vi "generate default name.vi"(11 "Info":T1={"Make"="Canon\u0000", "Model"="Canon PowerShot A495\u0000", "Orientation"=0, "Date"=timestamp(0 s since 1904-01-01), "Width"=0, "Height"=0, "Square?"=FALSE, "File Name"="Canon\u0000", "Extension"="Canon\u0000", "Valid?"=FALSE, "Path"=path "", "size"=0, "No Ext?"=FALSE, "prefix?"=FALSE, "Tag"="", "Name Type"=enum."Event Sufix", "Projection Type"="Canon\u0000"}) -> (1 "Model":string, 3 "default name":string)   [LabVIEW 2023, in "File Classes.lvlib" / "Picture File.lvclass"]
uses:
  Picture File.lvclass
  Controls/exif data cluster.ctl
  Controls/rename type enum.ctl
  <vilib>/gmath/NI_Gmath.lvlib
  File Classes.lvlib
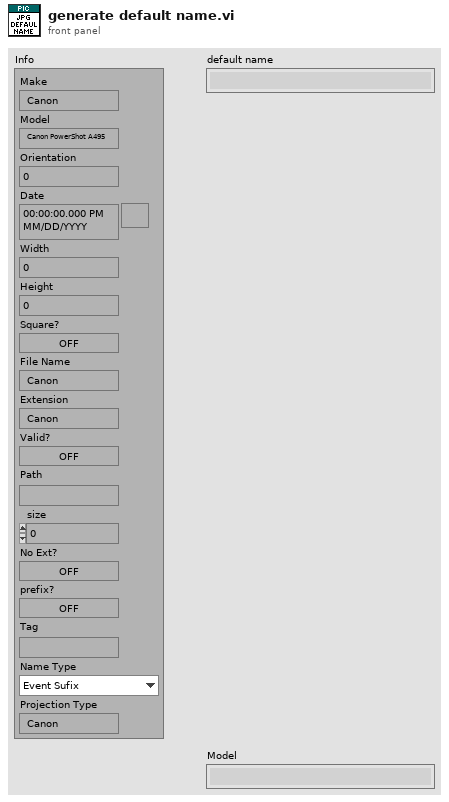
[diagram p1: front panel]
types:
  T1 = typedef "File Classes.lvlib/exif data cluster.ctl" = cluster{"Make":string, "Model":string, "Orientation":u16, "Date":timestamp, "Width":u16, "Height":u16, "Square?":bool, "File Name":string, "Extension":string, "Valid?":bool, "Path":path, "size":i64, "No Ext?":bool, "prefix?":bool, "Tag":string, "Name Type":T2, "Projection Type":string}
  T2 = typedef "File Classes.lvlib/rename type enum.ctl" = enum16{"Date & Time (Default)", "Model Sufix", "Event Sufix", "Model & Event Sufix"}
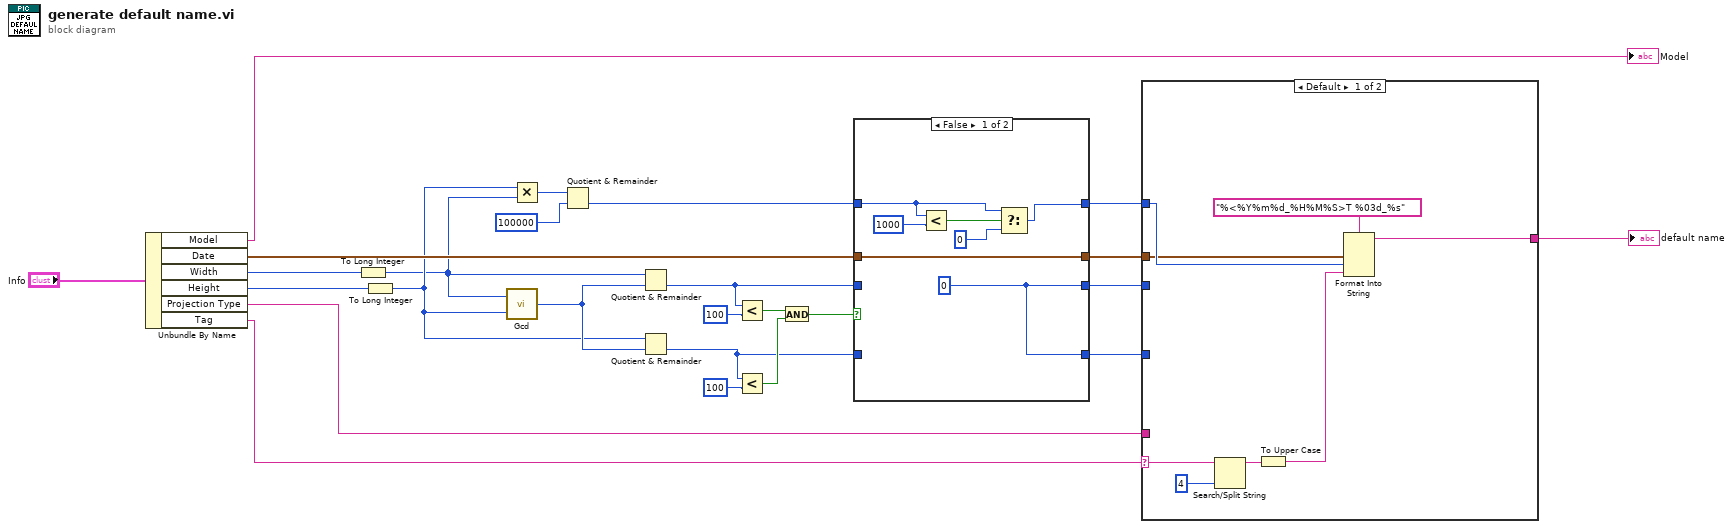
[diagram p0: block diagram]
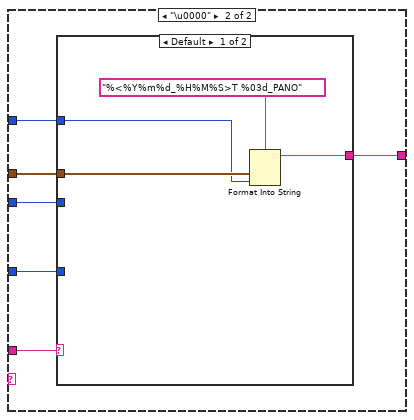
[diagram p2: hidden frame]
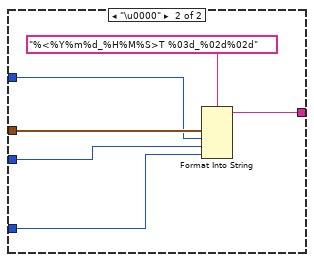
[diagram p3: hidden frame]
diagram:
  n1 = Unbundle By Name("Info") -> ("Model"=→"Model":string, "Date"=w23:timestamp, "Width"=w21:u16, "Height"=w20:u16, "Projection Type"=w2:string, "Tag"=w1:string)
  n2 = To Long Integer(number=w21) -> (32bit integer=w3:i32)
  n3 = To Long Integer(number=w20) -> (32bit integer=w12:i32)
  n4 = call <vilib>:"Gcd.vi"("y"=w12, "x"=w3) -> ("gcd(x,y)"=w15:i32)
  n5 = Multiply(x=w12, y=w3) -> (x*y=w14:i32)
  n6 = Quotient & Remainder(x=w14, y=100000) -> (floor(x/y)=w10:i32)  [unwired: 1 out]
  n7 = Quotient & Remainder(x=w3, y=w15) -> (floor(x/y)=w8:i32)  [unwired: 1 out]
  n8 = Quotient & Remainder(x=w12, y=w15) -> (floor(x/y)=w6:i32)  [unwired: 1 out]
  n9 = Less?(x=w8, y=100) -> (x < y?=w19:bool)
  n10 = Less?(x=w6, y=100) -> (x < y?=w18:bool)
  n11 = And(x=w19, y=w18) -> (x .and. y?=w11:bool)
  n12 = case shown="False" w11 {
    tunnel: [w29 w33] -> w4
    tunnel: w10 -> [w28 w33]
    tunnel: [w32 w34] -> w9
    tunnel: w23 -> [w32 w34]
    tunnel: [w27 w36] -> w5
    tunnel: w8 -> [_ w36]
    tunnel: [w27 w35] -> w7
    tunnel: w6 -> [_ w35]
    frame False {
      w27 = 0
      n13 = Less?(x=w28, y=1000) -> (x < y?=w30:bool)
      n14 = Select(t=w28, s=w30, f=0) -> (s? t:f=w29:i32)
    }
    frame True {
    }
  }
  n15 = case shown="Default" w1 {
    selector: w1 -> [w40 _]
    tunnel: [w41 w50] -> w25
    tunnel: w9 -> [w42 w49]
    tunnel: w7 -> [_ w48]
    tunnel: w5 -> [_ w47]
    tunnel: w4 -> [w43 w46]
    tunnel: w2 -> [_ w45]
    frame Default {
      n16 = Search/Split String(string=w40, offset (0)=4) -> (substring before match=w38:string)  [unwired: 1 in, 2 out]
      n17 = To Upper Case(1:w38) -> (0:w37:string)
      n18 = Format Into String(format string="%<%Y%m%d_%H%M%S>T %03d_%s", w42, w43, w37) -> (resulting string=w41:string)  [unwired: 2 in, 1 out]
    }
    frame "\u0000" {
      n19 = case shown="Default" w45 {
        tunnel: [w54 w60] -> w50
        tunnel: w49 -> [w52 w58]
        tunnel: w48 -> [_ w57]
        tunnel: w47 -> [_ w56]
        tunnel: w46 -> [w51 w55]
        frame Default {
          n20 = Format Into String(format string="%<%Y%m%d_%H%M%S>T %03d_PANO", w52, w51) -> (resulting string=w54:string)  [unwired: 2 in, 1 out]
        }
        frame "\u0000" {
          n21 = Format Into String(format string="%<%Y%m%d_%H%M%S>T %03d_%02d%02d", w58, w55, w56, w57) -> (resulting string=w60:string)  [unwired: 2 in, 1 out]
        }
      }
    }
  }
  "default name" <- w25
